vi "LLP Packet Generation Loop.vi"(0 "fpga interface in":refnum<k20>, 1 "'stop' notifier":refnum<notifier>, 5 "serial channels":string[](array[string]), 7 "source file paths":T1[](array[typedef]), 11 "error in":errorcluster) -> (15 "error out":errorcluster)   [LabVIEW 2023, in "GettingStarted_Gen_148X_Host.lvlib"]
uses:
  GettingStarted_Gen_148X_Host.lvlib
  Types/Channel Source File Paths.ctl
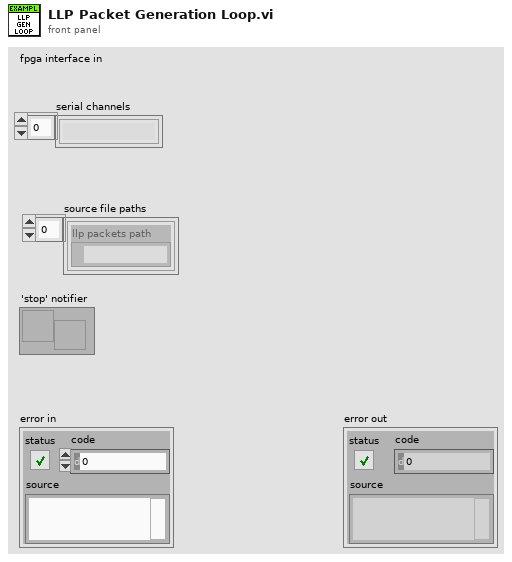
[diagram p1: front panel]
types:
  T1 = typedef "GettingStarted_Gen_148X_Host.lvlib/Channel Source File Paths.ctl" = cluster{"llp packets path":path}
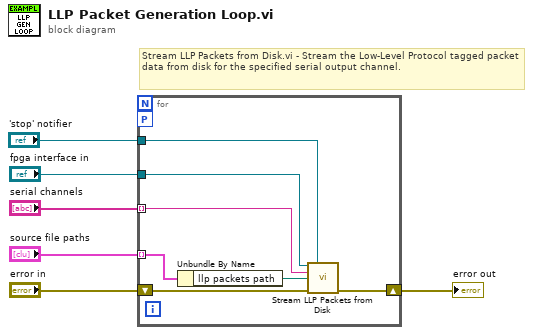
[diagram p0: block diagram]
diagram:
  # "Stream LLP Packets from Disk.vi - Stream the Low-Level Protocol tagged packet data from disk for the specified serial output channel."
  n1 = for {
    tunnel: "serial channels" -> [w7] mode=indexing
    tunnel: "fpga interface in" -> [w12]
    shift-right: [w10] -> w3
    shift-left: "error in" -> [w9]
    tunnel: "source file paths" -> [w13] mode=indexing
    workers-P: _ -> [_]
    tunnel: "'stop' notifier" -> [w11]
    n2 = Unbundle By Name(w13) -> ("llp packets path"=w8:path)
    n3 = call "Stream LLP Packets from Disk.vi"("fpga interface in"=w12, "'stop' notifier"=w11, "serial output channel"=w7, "llp data file path"=w8, "error in (no error)"=w9) -> ("error out"=w10:errorcluster)  [unwired: 9 in, 1 out]
  }
  "error out" <- w3
